vi "Split String.vi"(6 "Delimiter In":string, 9 "String In":string) -> (1 "String Array Out":string[](array[string]))   [LabVIEW 2026]
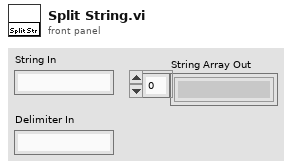
[diagram p1: front panel]
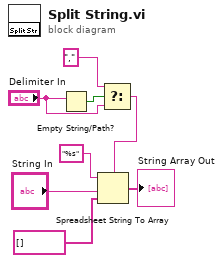
[diagram p0: block diagram]
diagram:
  n1 = Empty String/Path?(string/path="Delimiter In") -> (empty?=w2:bool)
  n2 = Select(t=",", s=w2, f="Delimiter In") -> (s? t:f=w4:string)
  n3 = Spreadsheet String To Array(delimiter (Tab)=w4, format string="%s", spreadsheet string="String In", array type (2D Dbl)=string[] []) -> (array=→"String Array Out":string[])
